vi "Write configure.vi"(8 "error in (no error)":errorcluster caption="错误输入（无错误）") -> (0 "错误输出":errorcluster)   [LabVIEW 2016, in "Alarm interface.lvlib"]
uses:
  Alarm interface.lvlib
  <vilib>/Utility/config.llb/NI_LVConfig.lvlib
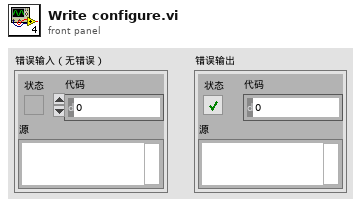
[diagram p1: front panel]
types:
  T1 = typedef "NI_LVConfig.lvlib/Config Data RefNum.ctl" = refnum<k1>
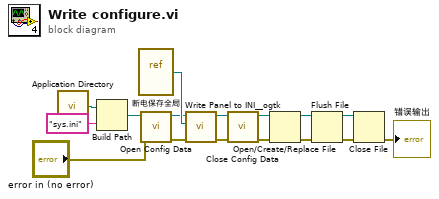
[diagram p0: block diagram]
diagram:
  n1 = call <vilib>:"Application Directory.vi"() -> ("Application Directory"=w14:path)
  n2 = Build Path(base path=w14, name or relative path="sys.ini" ("名称或相对路径")) -> (appended path=w15:path)
  n3 = vi-ref "断电保存全局.vi"() -> (w13:refnum<vi>)
  n4 = call <vilib>:"Open Config Data.vi"("error in (no error)"="error in (no error)", "configuration file path"=w15) -> ("error out"=w10:errorcluster, "refnum"=w12:T1)  [unwired: 7 in, 1 out]
  n5 = call <userlib>:"Write Panel to INI__ogtk.vi"("error in (no error)"=w10, "VI ref"=w13, "refnum"=w12) -> ("error out"=w9:errorcluster, "refnum out"=w11:T1)  [unwired: 7 in]
  n6 = call <vilib>:"Close Config Data.vi"("error in (no error)"=w9, "refnum"=w11) -> ("error out"=w4:errorcluster, "file path"=w3:path)  [unwired: 8 in]
  n7 = Open/Create/Replace File(file path (use dialog)=w3, error in=w4) -> (refnum out=w7:refnum<file>, error out=w8:errorcluster)  [unwired: 4 in, 1 out]
  n8 = Flush File(refnum=w7, error in=w8) -> (refnum out=w6:refnum<file>, error out=w5:errorcluster)
  n9 = Close File(refnum=w6, error in=w5) -> (error out=→"错误输出":errorcluster)  [unwired: 1 out]
